vi "Get Sciscan Frame.vi"(8 "error in (no error)":errorcluster, 11 "GFG reference":refnum<vi>) -> (0 "error out":errorcluster, 2 "image refs out":T2, 3 "GFG reference":refnum<vi>)   [LabVIEW 2012, in "Sciscan Scope Daemon.lvlib"]
uses:
  <vilib>/vision/Image Controls.llb/IMAQ Image.ctl
  Sciscan Scope Daemon.lvlib
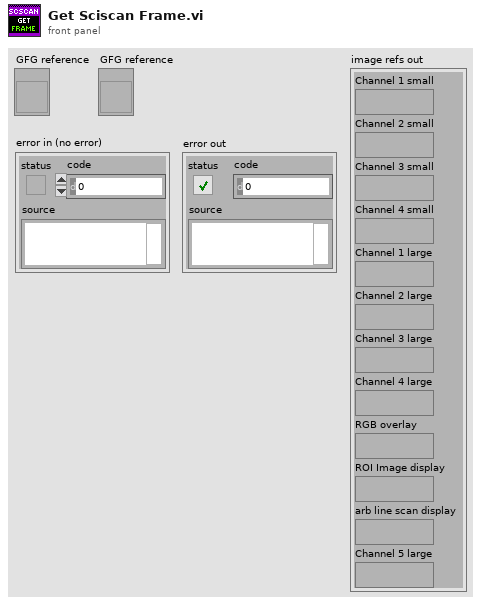
[diagram p1: front panel]
types:
  T1 = typedef "IMAQ Image.ctl" = refnum<image>
  T2 = cluster{"Channel 1 small":T1, "Channel 2 small":T1, "Channel 3 small":T1, "Channel 4 small":T1, "Channel 1 large":T1, "Channel 2 large":T1, "Channel 3 large":T1, "Channel 4 large":T1, "RGB overlay":T1, "ROI Image display":T1, "arb line scan display":T1, "Channel 5 large":T1}
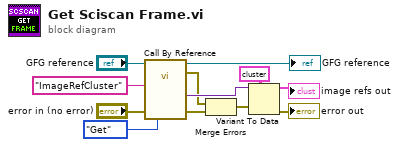
[diagram p0: block diagram]
diagram:
  n1 = call-by-ref "?"(reference="GFG reference", "Variable Name in"="ImageRefCluster", "error in (no error)"="error in (no error)", "Action"=enum16{"Init", "Set", "Get", "Clear"}."Get") -> (reference out=→"GFG reference":refnum<vi>, error out=w7:errorcluster, "Variant Out"=w9:variant, 19:"error out"=w6:errorcluster)  [unwired: 11 in, 5 out]
  n2 = Merge Errors(w7, w6) -> (w8:errorcluster)
  n3 = Variant To Data(error in=w8, type=T2 {"Channel 1 small"=refnum, "Channel 2 small"=refnum, "Channel 3 small"=refnum, "Channel 4 small"=refnum, "Channel 1 large"=refnum, "Channel 2 large"=refnum, "Channel 3 large"=refnum, "Channel 4 large"=refnum, "RGB overlay"=refnum, "ROI Image display"=refnum, "arb line scan display"=refnum, "Channel 5 large"=refnum} ("Image Refs Out"), Variant=w9) -> (data=→"image refs out":T2, error out=→"error out":errorcluster)
